vi "ControlMotores_sub.vi"(9 "Motores 2+3 (Eje x) 2":u32, 10 "Motores 2+3 (Eje x)":u32, 11 "Motor 1 (Eje z)":u32) -> (0 "error out":errorcluster)   [LabVIEW 2012]
uses:
  <vilib>/LabVIEW Interface for Arduino/LabVIEW Interface for Arduino.lvlib
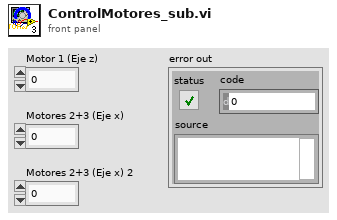
[diagram p1: front panel]
types:
  T1 = typedef "LabVIEW Interface for Arduino.lvlib/Arduino Resource.ctl" = cluster{"VISA resource":refnum<visa-resource-name>, "Board Type":T2, "Connection Type":enum8{"USB / Serial"}, "Bytes Per Packet (15)":u8}
  T2 = typedef "LabVIEW Interface for Arduino.lvlib/Board Type.ctl" = enum16{"Uno", "Dimuelanove w/Atmega 328", "Mega 2560"}
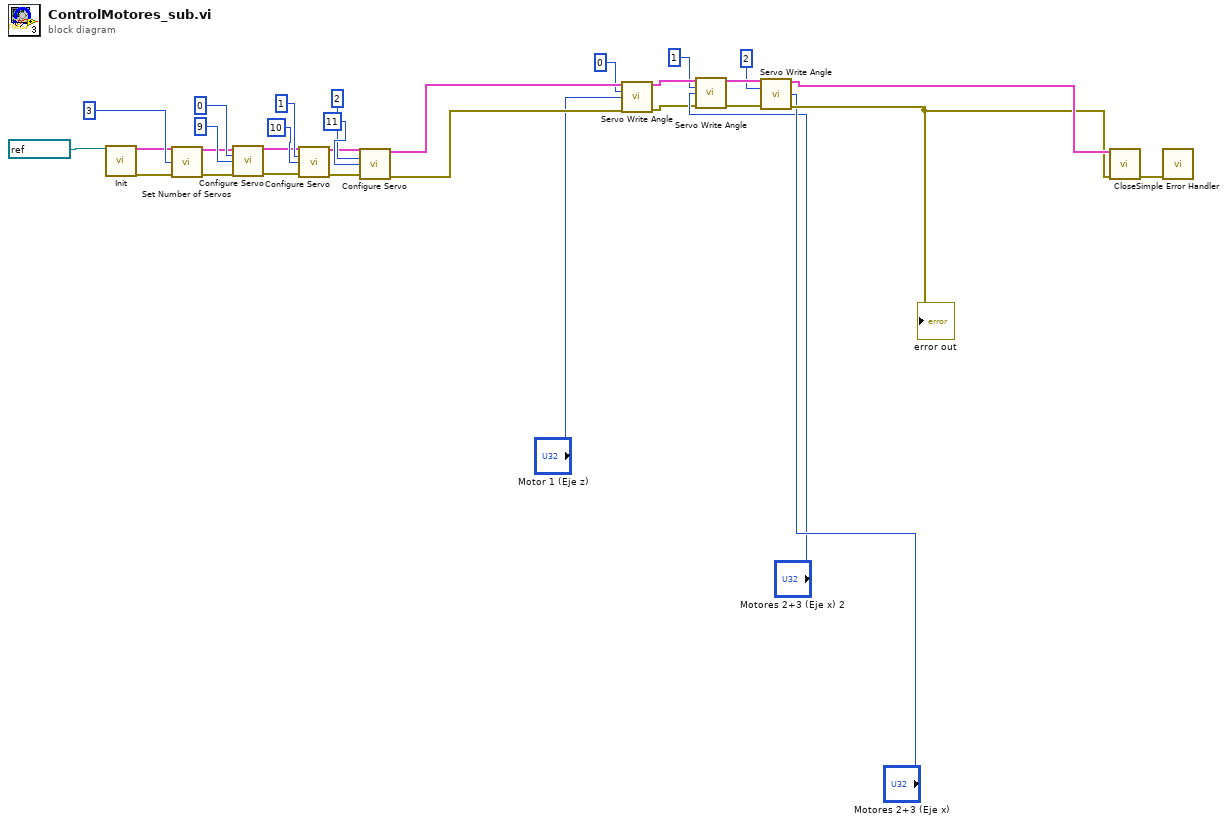
[diagram p0: block diagram]
diagram:
  n1 = call <vilib>:"Init.vi"("VISA resource"=refnum<visa-resource-name> "COM4") -> ("Arduino Resource"=w8:T1, "error out"=w1:errorcluster)  [unwired: 17 in]
  n2 = call <vilib>:"Set Number of Servos.vi"("Arduino Resource"=w8, "Number Of Servos (1)"=u8 3 ("Servo Number"), "error in"=w1) -> ("Arduino Resource"=w2:T1, "error out"=w3:errorcluster)  [unwired: 11 in]
  n3 = call <vilib>:"Configure Servo.vi"("Arduino Resource"=w2, "Servo Number (0)"=u8 0 ("Servo Number"), "DIO Pin (2)"=u8 9 ("Servo Number"), "error in"=w3) -> ("Arduino Resource"=w12:T1, "error out"=w10:errorcluster)  [unwired: 10 in]
  n4 = call <vilib>:"Configure Servo.vi"("Arduino Resource"=w12, "Servo Number (0)"=u8 1 ("Servo Number"), "DIO Pin (2)"=u8 10 ("Servo Number"), "error in"=w10) -> ("Arduino Resource"=w13:T1, "error out"=w11:errorcluster)  [unwired: 10 in]
  n5 = call <vilib>:"Configure Servo.vi"("Arduino Resource"=w13, "Servo Number (0)"=u8 2 ("Servo Number"), "DIO Pin (2)"=u8 11 ("Servo Number"), "error in"=w11) -> ("Arduino Resource"=w28:T1, "error out"=w29:errorcluster)  [unwired: 10 in]
  n6 = call <vilib>:"Servo Write Angle.vi"("Arduino Resource"=w28, "Servo Number"=u8 0, "Angle (Degrees)"="Motor 1 (Eje z)", "error in"=w29) -> ("Arduino Resource"=w21:T1, "error out"=w23:errorcluster)  [unwired: 10 in]
  n7 = call <vilib>:"Servo Write Angle.vi"("Arduino Resource"=w21, "Servo Number"=u8 1, "Angle (Degrees)"="Motores 2+3 (Eje x) 2", "error in"=w23) -> ("Arduino Resource"=w22:T1, "error out"=w24:errorcluster)  [unwired: 10 in]
  n8 = call <vilib>:"Servo Write Angle.vi"("Arduino Resource"=w22, "Servo Number"=u8 2, "Angle (Degrees)"="Motores 2+3 (Eje x)", "error in"=w24) -> ("Arduino Resource"=w31:T1, "error out"=w30:errorcluster)  [unwired: 10 in]
  "error out" <- w30
  n9 = call <vilib>:"Close.vi"("Arduino Resource"=w31, "error in"=w30) -> ("error out"=w7:errorcluster)  [unwired: 13 in]
  n10 = call <vilib>:"Simple Error Handler.vi"("error in (no error)"=w7) -> ()  [unwired: 4 in, 5 out]
